vi "Rename Chassis and All Connected Modules.vi"(8 "error in (no error)":errorcluster, 9 "new chassis name in":string, 10 "chassis name":refnum<k21>, 11 "session in":refnum<k21>) -> (0 "error out":errorcluster, 1 "new names of connected modules":refnum<k21>[](array[refnum]), 2 "new chassis name out":refnum<k21>, 3 "session out":refnum<k21>)   [LabVIEW 2020, in "SLSC.lvlib"]
doc: "Renames the chassis and all modules that connect to the chassis."
uses:
  <vilib>/SLSC/SLSC.lvlib
  <resource>/objmgr/slsc.rc
panel:
  out "names of connected modules":refnum<k21>[](array[refnum])
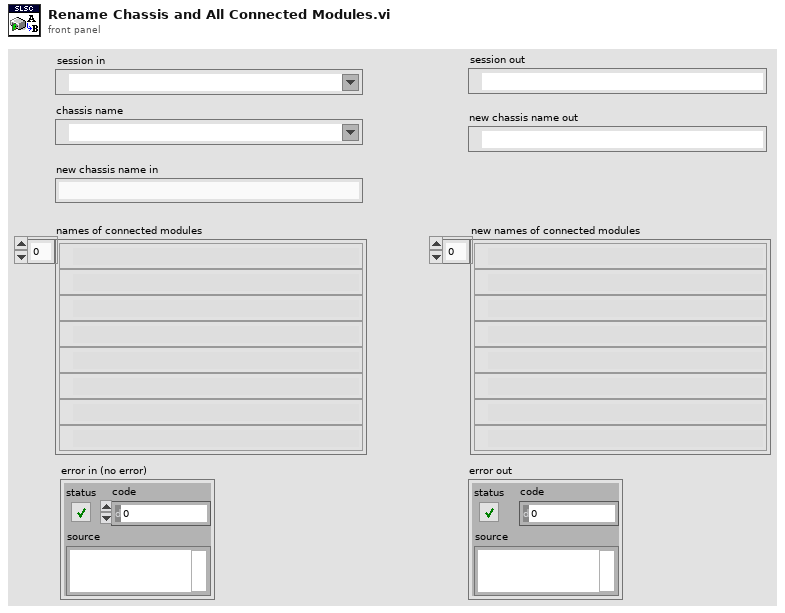
[diagram p1: front panel]
types:
  T1 = enum16{"Rename Modules", "Rename Chassis", "Wait for Chassis", "Wait for Modules"}[]
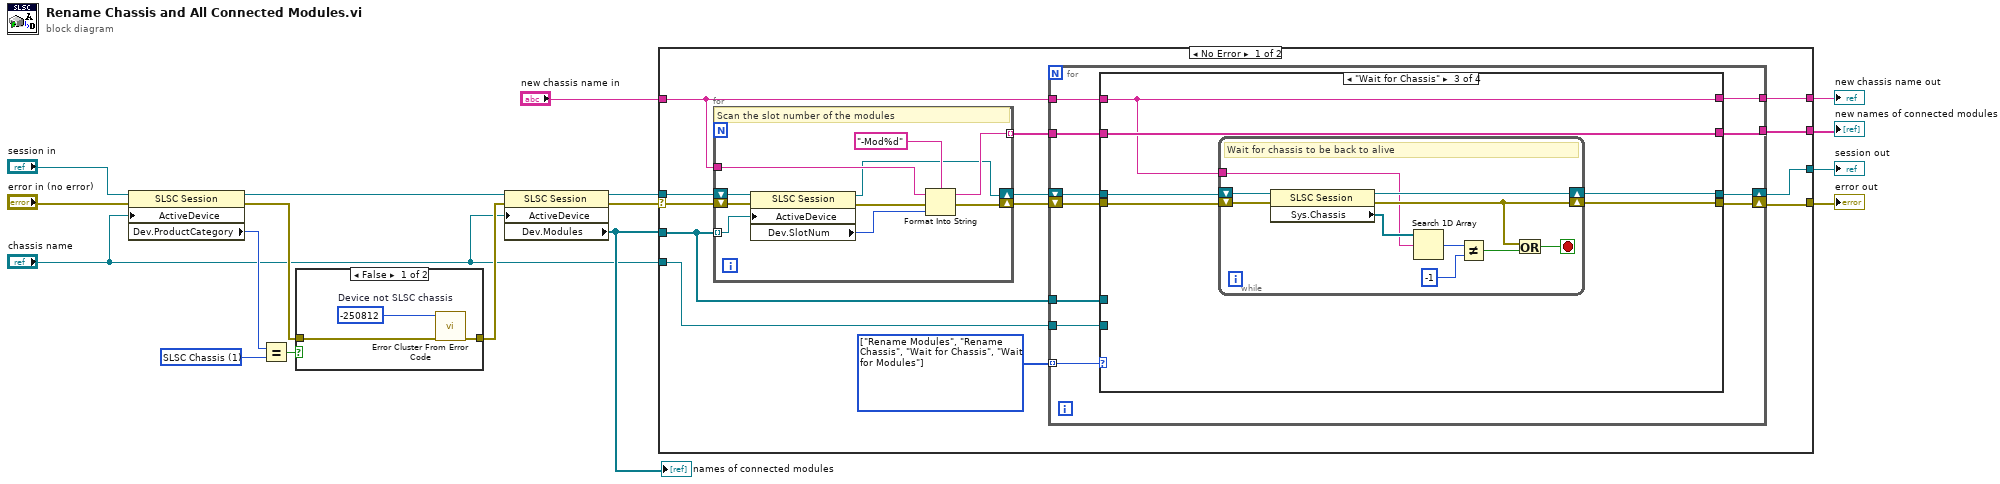
[diagram p0: block diagram]
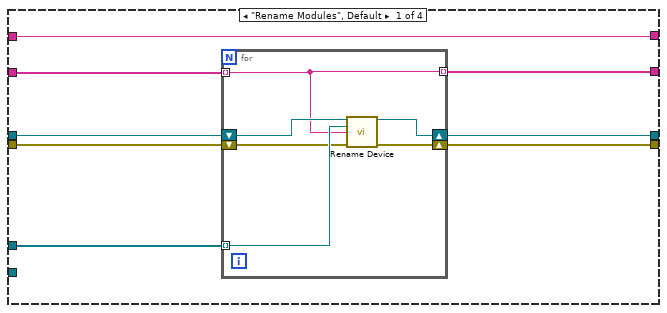
[diagram p2: hidden frame]
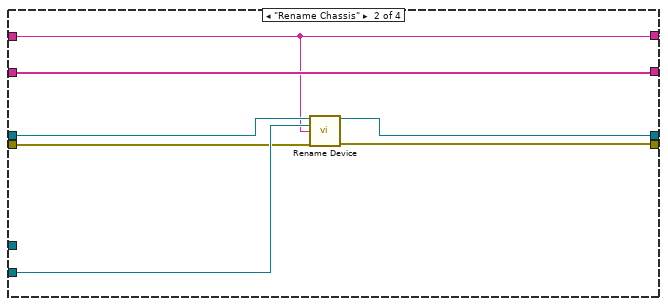
[diagram p3: hidden frame]
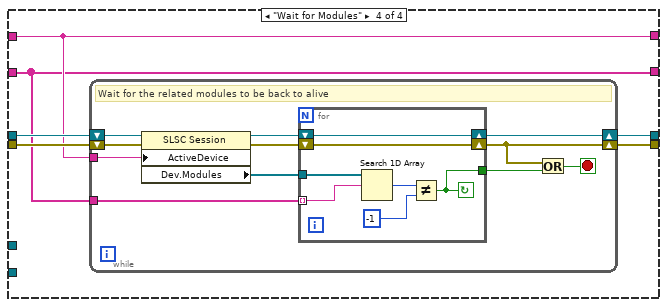
[diagram p4: hidden frame]
diagram:
  w16 = 1 items=["Unknown", "SLSC Chassis", "SLSC Module"] ("Dev.ProductCategory")
  n1 = property class="SLSC Session"(reference="session in", error in="error in (no error)", "ActiveDevice"="chassis name") -> (reference out=w13:refnum<k21>, error out=w14:errorcluster, "Dev.ProductCategory"=w10:i32)
  n2 = Equal?(x=w10, y=w16) -> (x = y?=w17:bool)
  n3 = case shown="False" w17 {
    tunnel: [w19 w21] -> w15
    tunnel: w14 -> [w18 w21]
    frame False {
      w20 = -250812  # Device not SLSC chassis
      n4 = call <vilib>:"Error Cluster From Error Code.vi"("error in (no error)"=w18, "error code (0)"=w20) -> ("error out"=w19:errorcluster)  [unwired: 7 in]
    }
    frame True {
    }
  }
  n5 = property class="SLSC Session"(reference=w13, error in=w15, "ActiveDevice"="chassis name") -> (reference out=w9:refnum<k21>, error out=w8:errorcluster, "Dev.Modules"=w6:refnum<k21>[])
  "names of connected modules" <- w6
  n6 = case shown="No Error" w8 {
    selector: w8 -> [w34 w117]
    tunnel: w6 -> [w32 _]
    tunnel: "new chassis name in" -> [w24 _]
    tunnel: "chassis name" -> [w25 _]
    tunnel: w9 -> [w33 w118]
    tunnel: [w22 _] -> w2
    tunnel: [w23 _] -> w1
    tunnel: [w27 w118] -> w3
    tunnel: [w26 w117] -> w4
    frame No Error {
      w30 = T1 [enum."Rename Modules", enum."Rename Chassis", enum."Wait for Chassis", enum."Wait for Modules"] items=["Rename Modules", "Rename Chassis", "Wait for Chassis", "Wait for Modules"]
      n7 = for {
        tunnel: w32 -> [w115] mode=indexing
        tunnel: w24 -> [w112]
        tunnel: [w110] -> w31 mode=indexing
        shift-right: [w109] -> w29
        shift-left: w34 -> [w116]
        shift-right: [w108] -> w28
        shift-left: w33 -> [w114]
        # "Scan the slot number of the modules"
        n8 = property class="SLSC Session"(reference=w114, error in=w116, "ActiveDevice"=w115) -> (reference out=w108:refnum<k21>, error out=w113:errorcluster, "Dev.SlotNum"=w107:u32)
        n9 = Format Into String(format string="-Mod%d", initial string=w112, error in=w113, w107) -> (resulting string=w110:string, error out=w109:errorcluster)
      }
      n10 = for {
        tunnel: w30 -> [w45] mode=indexing
        shift-right: [w42] -> w27
        shift-left: w28 -> [w44]
        tunnel: w31 -> [w40]
        tunnel: w32 -> [w39]
        tunnel: [w38] -> w22
        tunnel: w25 -> [w37]
        tunnel: w24 -> [w36]
        tunnel: [w35] -> w23
        shift-right: [w41] -> w26
        shift-left: w29 -> [w43]
        n11 = case shown="\"Wait for Chassis\"" w45 {
          tunnel: w44 -> [w53 w66 w72 w86]
          tunnel: w39 -> [w52 _ _ _]
          tunnel: w40 -> [w51 w61 w70 w83]
          tunnel: w43 -> [w50 w64 w71 w85]
          tunnel: [w49 w63 w69 w88] -> w42
          tunnel: [w48 w62 w68 w87] -> w41
          tunnel: [w47 w61 w70 w83] -> w38
          tunnel: w37 -> [_ w65 _ _]
          tunnel: w36 -> [w46 w60 w67 w84]
          tunnel: [w46 w60 w67 w84] -> w35
          frame "Rename Modules", Default {
            n12 = for {
              tunnel: w52 -> [w58] mode=indexing
              tunnel: w51 -> [w54] mode=indexing
              tunnel: [w54] -> w47 mode=indexing
              shift-right: [w55] -> w48
              shift-left: w50 -> [w57]
              shift-right: [w56] -> w49
              shift-left: w53 -> [w59]
              n13 = call <vilib>:"Rename Device.vi"("session in"=w59, "device"=w58, "new device name"=w54, "error in (no error)"=w57) -> ("session out"=w56:refnum<k21>, "error out"=w55:errorcluster)  [unwired: 10 in]
            }
          }
          frame "Rename Chassis" {
            n14 = call <vilib>:"Rename Device.vi"("session in"=w66, "device"=w65, "new device name"=w60, "error in (no error)"=w64) -> ("session out"=w63:refnum<k21>, "error out"=w62:errorcluster)  [unwired: 10 in]
          }
          frame "Wait for Chassis" {
            n15 = while {
              tunnel: w67 -> [w73]
              shift-right: [w78] -> w68
              shift-left: w71 -> [w75]
              shift-right: [w76] -> w69
              shift-left: w72 -> [w74]
              stop <- w77 stop-if-true
              # "Wait for chassis to be back to alive"
              n16 = property class="SLSC Session"(reference=w74, error in=w75) -> (reference out=w76:refnum<k21>, error out=w78:errorcluster, "Sys.Chassis"=w82:refnum<k21>[])
              n17 = Search 1D Array(1D array=w82, element=w73) -> (index of element=w81:i32)  [unwired: 1 in]
              n18 = Not Equal?(x=w81, y=-1) -> (x != y?=w79:bool)
              n19 = Or(x=w78, y=w79) -> (x .or. y?=w77:bool)
            }
          }
          frame "Wait for Modules" {
            n20 = while {
              shift-right: [w94] -> w87
              shift-left: w85 -> [w98]
              tunnel: w83 -> [w91]
              tunnel: w84 -> [w89]
              shift-right: [w93] -> w88
              shift-left: w86 -> [w99]
              stop <- w97 stop-if-true
              # "Wait for the related modules to be back to alive"
              n21 = property class="SLSC Session"(reference=w99, error in=w98, "ActiveDevice"=w89) -> (reference out=w96:refnum<k21>, error out=w95:errorcluster, "Dev.Modules"=w92:refnum<k21>[])
              n22 = for {
                tunnel: w91 -> [w102] mode=indexing
                tunnel: w92 -> [w103]
                tunnel: [w100] -> w90
                shift-right: [w104] -> w93
                shift-left: w96 -> [w104]
                shift-right: [w101] -> w94
                shift-left: w95 -> [w101]
                stop <- w100 continue-if-true
                n23 = Search 1D Array(1D array=w103, element=w102) -> (index of element=w106:i32)  [unwired: 1 in]
                n24 = Not Equal?(x=w106, y=-1) -> (x != y?=w100:bool)
              }
              n25 = Or(x=w94, y=w90) -> (x .or. y?=w97:bool)
            }
          }
        }
      }
    }
    frame Error {
    }
  }
  "new names of connected modules" <- w2
  "new chassis name out" <- w1
  "session out" <- w3
  "error out" <- w4
